vi "InIt global.vi"(8 "error in":errorcluster) -> (0 "error out":errorcluster, 3 "out":string)   [LabVIEW 2009]
uses:
  Global/Global 1.vi
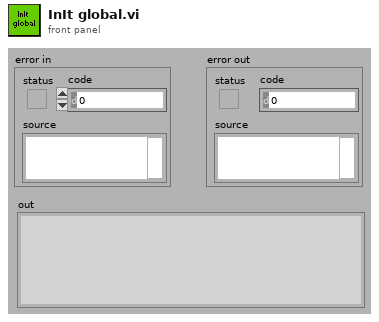
[diagram p1: front panel]
types:
  T1 = cluster{"serial number":string, "Part number":string, "Revision letter ":string, "Revision counter":string, "Manufature":string, "Year Week":string}
  T2 = cluster{"People":string, "product  number":string, "Test time":string, "VHeatFuse_noload":string, "VHeatFuse_load":string, "VoverrideDiode":string, "Test firmware upload via X1":string, "TemperAddress":string, "Troom":string, "TLCU":string, "Adjustment factor":string, "MeasuredFreq":string, "I2C communication":string, "Light-emitting diode on Z2":string, "Battery warning/inhibit":string, "Reset by IC10":string, "External EEPROM":string, "RFID card detection and reading RFID":string, "Production parameters in internal EEPROM":string, "Current consumption in sleep mode":string, "Application and database upload":string, "Test result":string, "Table head[22]":string, "Table head[23]":string}
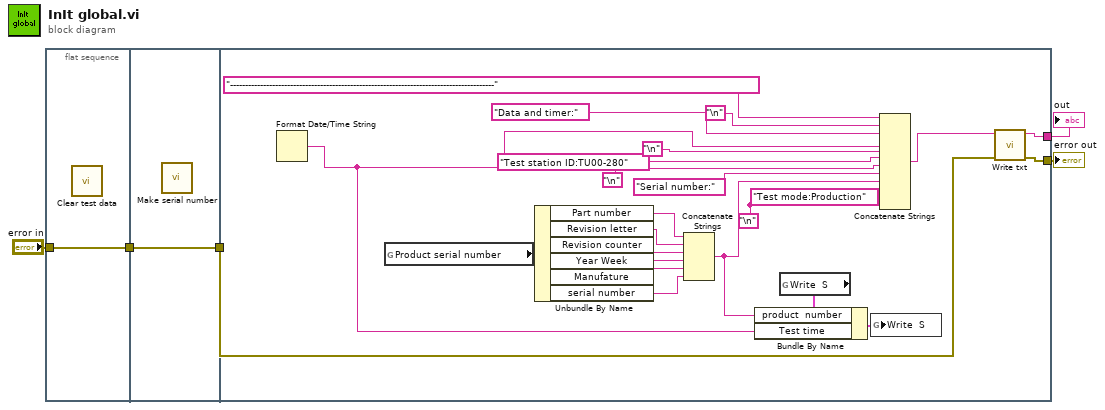
[diagram p0: block diagram]
diagram:
  n1 = flat-sequence {
    tunnel: "error in" -> [w6]
    tunnel: [w6] -> w1
    tunnel: [w7] -> w5
    tunnel: w1 -> [w7]
    tunnel: [w19] -> w3
    tunnel: w5 -> [w18]
    tunnel: [w17] -> w2
    frame #0 {
      n2 = call "Clear test data.vi"() -> ()  [unwired: 12 out]
    }
    frame #1 {
      n3 = call "Make serial number.vi"() -> ()  [unwired: 12 out]
    }
    frame #2 {
      w13 = "\n"
      n4 = Format Date/Time String() -> (date/time string=w8:string)  [unwired: 3 out]
      n5 = global read "Global 1.vi" "Product serial number"() -> (w26:T1)
      n6 = Unbundle By Name(w26) -> ("Part number"=w25:string, "Revision letter"=w24:string, "Revision counter"=w23:string, "Year Week"=w22:string, "Manufature"=w21:string, "serial number"=w20:string)
      n7 = Concatenate Strings(w25, w24, w23, w22, w21, w20) -> (w9:string)
      n8 = global read "Global 1.vi" "Write  S"() -> (w11:T2)
      n9 = Bundle By Name(cluster=w11, "product  number"=w9, "Test time"=w8) -> (w10:T2)
      n10 = global write "Global 1.vi" "Write  S"(w10) -> ()
      n11 = Concatenate Strings("----------------------------------------------------------------------------------------", "\n", "Data and timer:" ("string"), w8, "\n", "Test station ID:TU00-280" ("string"), "\n", "Serial number:" ("string"), w9, w13, "Test mode:Production" ("string"), w13) -> (w31:string)
      n12 = call "Write txt.vi"("error in"=w18, "IN String"=w31) -> ("error out"=w19:errorcluster, "out"=w17:string)  [unwired: 8 out]
    }
  }
  "error out" <- w3
  "out" <- w2
